vi "Filter Shortcut Menu Activation Event.vi"(8 "error in (no error)":errorcluster, 10 "ShortcutMenuActivationMsg":refnum<class "ShortcutMenuActivationMsg.lvclass">, 11 "TestEventFilter in":refnum<class "TestEventFilter.lvclass">) -> (0 "error out":errorcluster, 1 "Discard?":bool, 3 "TestEventFilter out":refnum<class "TestEventFilter.lvclass">)   [LabVIEW 2020, in "TestViewables.lvlib" / "TestEventFilter.lvclass"]
uses:
  TestEventFilter.lvclass
  modules/mva-viewable/Source/ActorEvents/IEventAggregator Messages/ShortcutMenuActivationMsg/ShortcutMenuActivationMsg.lvclass
  TestEventFilter.lvclass/TestEventFilter.ctl
  modules/mva-viewable/Source/ActorEvents/IEventAggregator Messages/ShortcutMenuActivationMsg/ShortcutMenuActivationMsg.lvclass/ShortcutMenuActivationMsg.ctl
  modules/mva-viewable/Source/ActorEvents/IEventAggregator Messages/ShortcutMenuActivationMsg/Accessors/Read MenuRef.vi
panel:
  # "No additional\nEvent Data"
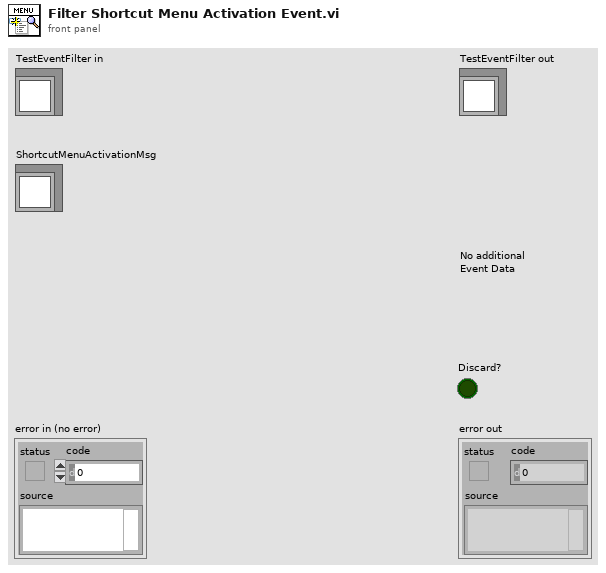
[diagram p1: front panel]
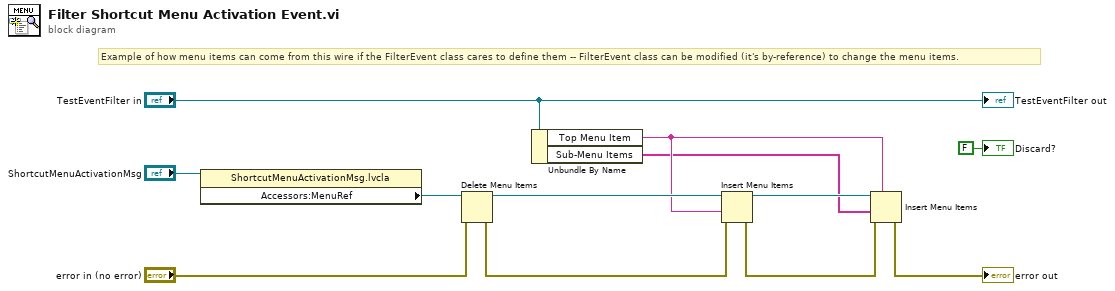
[diagram p0: block diagram]
diagram:
  # "Example of how menu items can come from this wire if the FilterEvent class cares to define them -- FilterEvent class can be modified (it's by-reference) to change the menu items."
  n1 = property class="ShortcutMenuActivationMsg.lvcla"(reference="ShortcutMenuActivationMsg") -> ("Accessors:MenuRef"=w4:refnum<k9>)  [unwired: 1 in, 2 out]
  n2 = Delete Menu Items(6:"error in (no error)", 9:w4) -> (0:w8:errorcluster, 3:w11:refnum<k9>)  [unwired: 2 in]
  n3 = Unbundle By Name("TestEventFilter in") -> ("Top Menu Item"=w2:string, "Sub-Menu Items"=w1:string[])
  n4 = Insert Menu Items(6:w8, 7:w2, 9:w11) -> (0:w7:errorcluster, 3:w12:refnum<k9>)  [unwired: 3 in, 1 out]
  n5 = Insert Menu Items(5:w2, 6:w7, 7:w1, 9:w12) -> (0:→"error out":errorcluster)  [unwired: 2 in, 2 out]
  "TestEventFilter out" <- "TestEventFilter in"
  "Discard?" <- FALSE ("Discard?")
